vi "filter control reference.vi"(8 "error in (no error)":errorcluster, 10 "Control label":string, 11 "VI (Caller)":refnum<vi>) -> (0 "error out":errorcluster, 2 "Control found":bool, 3 "Control ref":refnum<vi>)   [LabVIEW 2020, in "ui-testing.lvlib"]
uses:
  ui-testing.lvlib
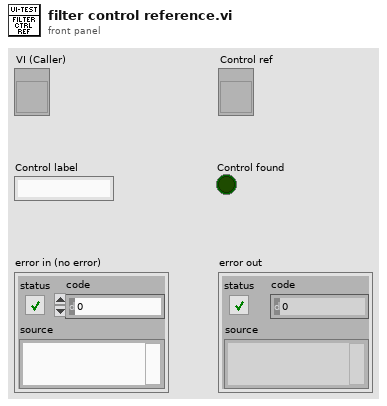
[diagram p1: front panel]
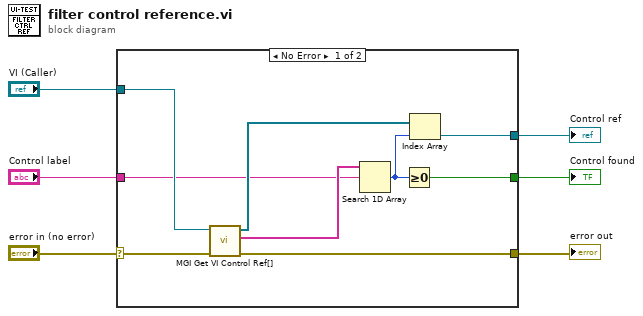
[diagram p0: block diagram]
diagram:
  n1 = case shown="No Error" "error in (no error)" {
    selector: "error in (no error)" -> [w14 _]
    tunnel: "VI (Caller)" -> [w15 _]
    tunnel: "Control label" -> [w10 _]
    tunnel: [w9 _] -> w3
    tunnel: [w8 _] -> w2
    tunnel: [w7 _] -> w1
    frame No Error {
      n2 = call <userlib>:"MGI Get VI Control Ref[].vi"("error in"=w14, "VI (Caller)"=w15) -> ("error out"=w9:errorcluster, "Control Label Chain[i]"=w11:string[], "Control[i]"=w12:refnum<vi>[])  [unwired: 6 in, 1 out]
      n3 = Search 1D Array(1D array=w11, element=w10) -> (index of element=w13:i32)  [unwired: 1 in]
      n4 = Greater Or Equal To 0?(x=w13) -> (x >= 0?=w8:bool)
      n5 = Index Array(array=w12, index=w13) -> (element=w7:refnum<vi>)
    }
    frame Error {
    }
  }
  "error out" <- w3
  "Control found" <- w2
  "Control ref" <- w1
